vi "WaitUntilExit.vi"(6 "Timeout(-1)":i32=-1, 8 "ErrorIn":errorcluster, 11 "YActor in":refnum<class "YActor.lvclass">) -> (0 "ErrorOut":errorcluster, 1 "Timeout":bool, 3 "YActor out":refnum<class "YActor.lvclass">)   [LabVIEW 2021, in "YActor.lvclass"]
uses:
  YActor.lvclass
  YActor.lvclass/YActor.ctl
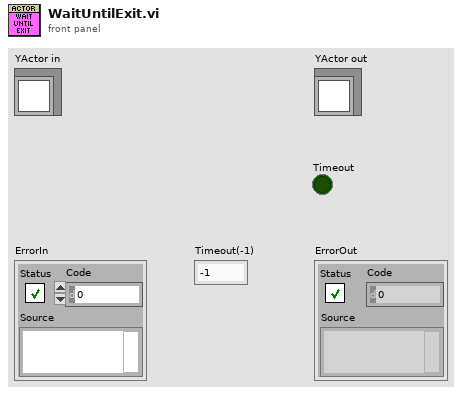
[diagram p1: front panel]
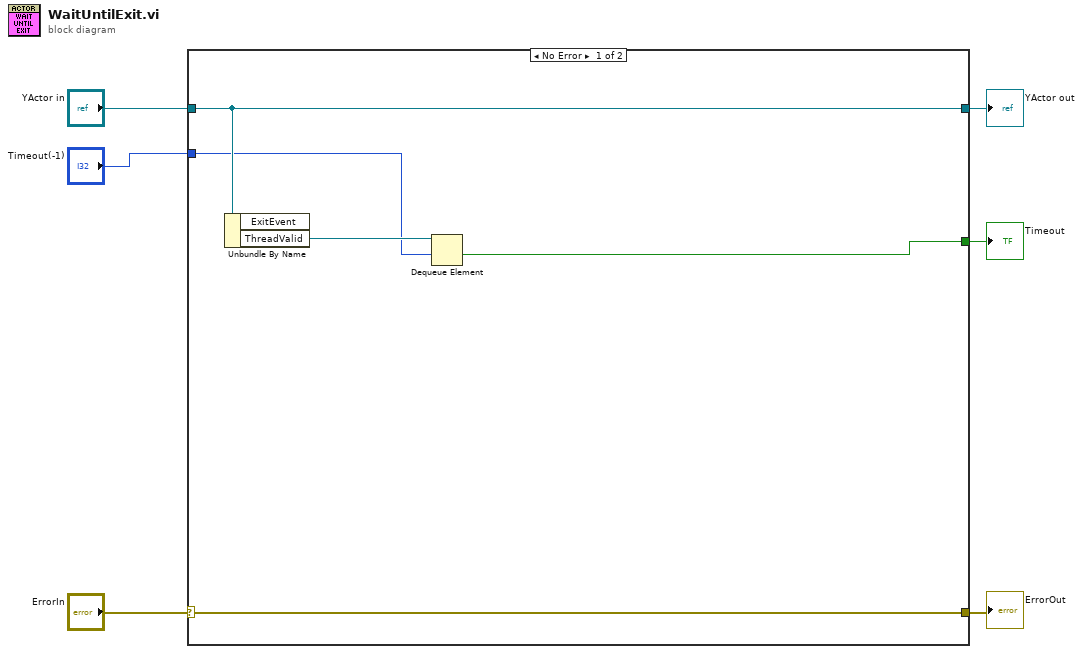
[diagram p0: block diagram]
diagram:
  n1 = case shown="No Error" "ErrorIn" {
    selector: "ErrorIn" -> [w11 w13]
    tunnel: [w11 w13] -> w5
    tunnel: [w10 w12] -> w3
    tunnel: "YActor in" -> [w10 w12]
    tunnel: "Timeout(-1)" -> [w8 _]
    tunnel: [w7 _] -> w1
    frame No Error {
      n2 = Unbundle By Name(w10) -> ("ThreadValid"=w9:refnum<queue>)  [unwired: 1 out]
      n3 = Dequeue Element(queue=w9, timeout in ms (-1)=w8) -> (timed out?=w7:bool)  [unwired: 1 in, 3 out]
    }
    frame Error {
    }
  }
  "ErrorOut" <- w5
  "YActor out" <- w3
  "Timeout" <- w1
